vi "Set Termination TTL.vi"(0 "Tosca in":refnum<class "Parameters.lvclass">, 5 "TTL":refnum<class "TTLController.lvclass">[](array[class]), 7 "stateIndex":i32, 9 "termIndex":i32, 11 "error in (no error)":errorcluster) -> (4 "Tosca out":refnum<class "Parameters.lvclass">, 15 "error out":errorcluster)   [LabVIEW 2015, in "Parameters.lvclass"]
uses:
  Parameters.lvclass
  TTL VIs/Control Classes/Base Class/TTLController.lvclass
  Parameters.lvclass/Parameters.ctl
  State/State.lvclass
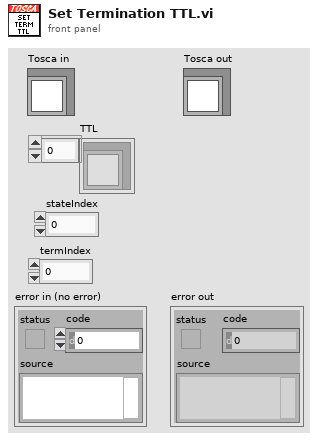
[diagram p1: front panel]
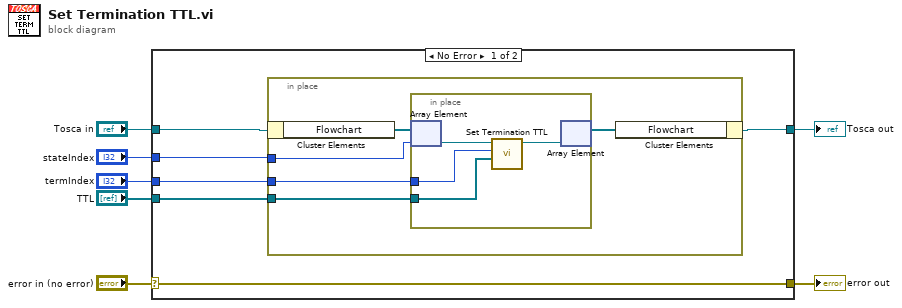
[diagram p0: block diagram]
diagram:
  n1 = case shown="No Error" "error in (no error)" {
    selector: "error in (no error)" -> [w13 w24]
    tunnel: [w13 w24] -> w6
    tunnel: [w11 w23] -> w4
    tunnel: "Tosca in" -> [w12 w23]
    tunnel: "stateIndex" -> [w10 _]
    tunnel: "termIndex" -> [w9 _]
    tunnel: "TTL" -> [w8 _]
    frame No Error {
      n2 = in-place {
        in-place-border: w10 -> [w17]
        in-place-border: w8 -> [w15]
        in-place-border: w9 -> [w14]
        n3 = in-place-cluster #1(w12) -> ("Flowchart"=w18:refnum<class "State.lvclass">[])
        n4 = in-place {
          in-place-border: w15 -> [w19]
          in-place-border: w14 -> [w20]
          n5 = in-place-array #2(w18, w17) -> (w21:refnum<class "State.lvclass">)
          n6 = call "Set Termination TTL.vi"("TTL"=w19, "termIndex"=w20, "State in"=w21) -> ("State out"=w22:refnum<class "State.lvclass">)  [unwired: 7 in, 1 out]
          n7 = in-place-array #2(w22) -> (w16:refnum<class "State.lvclass">[])  [unwired: 1 out]
        }
        n8 = in-place-cluster #1("Flowchart"=w16) -> (w11:refnum<class "Parameters.lvclass">)
      }
    }
    frame Error {
    }
  }
  "error out" <- w6
  "Tosca out" <- w4
